vi "GetNumericWithScaleReference.vi"(8 "error in":errorcluster, 11 "NumericWithScale in":refnum<class "NumericWithScale.lvclass">) -> (0 "error out":errorcluster, 1 "numeric with scale reference":refnum<vi>, 3 "NumericWithScale out":refnum<class "NumericWithScale.lvclass">)   [LabVIEW 2014, in "NumericWithScale.lvclass"]
uses:
  NumericWithScale.lvclass
  Generic/Generic.lvclass
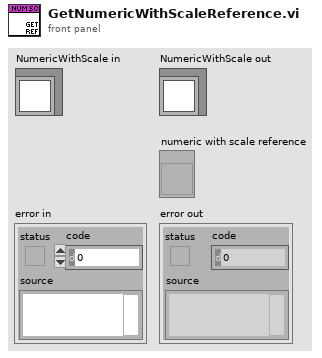
[diagram p1: front panel]
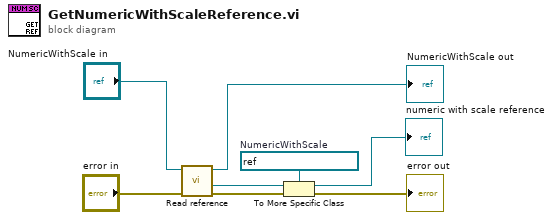
[diagram p0: block diagram]
diagram:
  w5 = refnum<vi> refnum  # NumericWithScale
  n1 = call "Read reference.vi"("error in"="error in", "GObject in"="NumericWithScale in") -> ("error out"=w6:errorcluster, "reference"=w7:refnum<vi>, "GObject out"=→"NumericWithScale out":refnum<class "NumericWithScale.lvclass">)  [unwired: 5 in]
  n2 = To More Specific Class(target class=w5, reference=w7, error in=w6) -> (specific class reference=→"numeric with scale reference":refnum<vi>, error out=→"error out":errorcluster)
